vi "Continuous CDF.vi"   [LabVIEW 2020, in "NI_Gmath.lvlib"]
doc: "Computes the continuous cumulative distribution function (CDF), or the probability that the random variate X, where X describes the selected distribution type, has a value less than or equal to <B>x</B>. You must manually select the polymorphic instance to use."
uses:
  <vilib>/gmath/NI_Gmath.lvlib
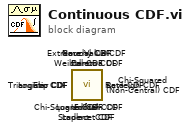
[diagram p0: block diagram]
diagram:
  n1 = call <vilib>:"Lognormal CDF.vi"() -> ()  [unwired: 10 in, 2 out]
  n2 = call <vilib>:"Pareto CDF.vi"() -> ()  [unwired: 10 in, 2 out]
  n3 = call <vilib>:"Logistic CDF.vi"() -> ()  [unwired: 10 in, 2 out]
  n4 = call <vilib>:"Chi-Squared (Non-Central) CDF.vi"() -> ()  [unwired: 10 in, 2 out]
  n5 = call <vilib>:"Laplace CDF.vi"() -> ()  [unwired: 10 in, 2 out]
  n6 = call <vilib>:"Extreme Value CDF.vi"() -> ()  [unwired: 10 in, 2 out]
  n7 = call <vilib>:"Weibull CDF.vi"() -> ()  [unwired: 10 in, 2 out]
  n8 = call <vilib>:"Uniform CDF.vi"() -> ()  [unwired: 10 in, 2 out]
  n9 = call <vilib>:"Triangular CDF.vi"() -> ()  [unwired: 10 in, 2 out]
  n10 = call <vilib>:"Student t CDF.vi"() -> ()  [unwired: 9 in, 3 out]
  n11 = call <vilib>:"Rayleigh CDF.vi"() -> ()  [unwired: 10 in, 2 out]
  n12 = call <vilib>:"Normal CDF.vi"() -> ()  [unwired: 10 in, 2 out]
  n13 = call <vilib>:"Gamma CDF.vi"() -> ()  [unwired: 10 in, 2 out]
  n14 = call <vilib>:"F CDF.vi"() -> ()  [unwired: 10 in, 2 out]
  n15 = call <vilib>:"Exp CDF.vi"() -> ()  [unwired: 10 in, 2 out]
  n16 = call <vilib>:"Chi-Squared CDF.vi"() -> ()  [unwired: 10 in, 2 out]
  n17 = call <vilib>:"Cauchy CDF.vi"() -> ()  [unwired: 10 in, 2 out]
  n18 = call <vilib>:"Beta CDF.vi"() -> ()  [unwired: 10 in, 2 out]
